vi "score sorter.vi"(11 "array of cluster":cluster{"Score":dbl, "Student ID":dbl}[](array[cluster])=[{"Score"=0.0, "Student ID"=1.0}, {"Score"=0.0, "Student ID"=2.0}, {"Score"=0.0, "Student ID"=3.0}, {"Score"=0.0, "Student ID"=4.0}, {"Score"=0.0, "Student ID"=5.0}, {"Score"=0.0, "Student ID"=6.0}, {"Score"=0.0, "Student ID"=7.0}, {"Score"=0.0, "Student ID"=8.0}, {"Score"=0.0, "Student ID"=9.0}, {"Score"=0.0, "Student ID"=10.0}, {"Score"=0.0, "Student ID"=11.0}, {"Score"=0.0, "Student ID"=12.0}, {"Score"=0.0, "Student ID"=13.0}, {"Score"=0.0, "Student ID"=14.0}, {"Score"=0.0, "Student ID"=15.0}, {"Score"=0.0, "Student ID"=16.0}, {"Score"=0.0, "Student ID"=17.0}, {"Score"=0.0, "Student ID"=18.0}, {"Score"=0.0, "Student ID"=19.0}, {"Score"=0.0, "Student ID"=20.0}, {"Score"=0.0, "Student ID"=21.0}, {"Score"=0.0, "Student ID"=22.0}, {"Score"=0.0, "Student ID"=23.0}, {"Score"=0.0, "Student ID"=24.0}, {"Score"=0.0, "Student ID"=25.0}, {"Score"=0.0, "Student ID"=26.0}, {"Score"=0.0, "Student ID"=27.0}, {"Score"=0.0, "Student ID"=28.0}, {"Score"=0.0, "Student ID"=29.0}, {"Score"=0.0, "Student ID"=30.0}, {"Score"=0.0, "Student ID"=31.0}, {"Score"=0.0, "Student ID"=32.0}, {"Score"=0.0, "Student ID"=33.0}, {"Score"=0.0, "Student ID"=34.0}, {"Score"=0.0, "Student ID"=35.0}, {"Score"=0.0, "Student ID"=36.0}, {"Score"=0.0, "Student ID"=37.0}, {"Score"=0.0, "Student ID"=38.0}, {"Score"=0.0, "Student ID"=39.0}, {"Score"=0.0, "Student ID"=40.0}, {"Score"=0.0, "Student ID"=41.0}, {"Score"=0.0, "Student ID"=42.0}, {"Score"=0.0, "Student ID"=43.0}, {"Score"=0.0, "Student ID"=44.0}, {"Score"=0.0, "Student ID"=45.0}, {"Score"=0.0, "Student ID"=46.0}, {"Score"=0.0, "Student ID"=47.0}, {"Score"=0.0, "Student ID"=48.0}, {"Score"=0.0, "Student ID"=49.0}, {"Score"=0.0, "Student ID"=50.0}]) -> (3 "sorted by score":cluster{"Score":dbl, "Student ID":dbl}[](array[cluster])=[{"Score"=0.0, "Student ID"=1.0}, {"Score"=0.0, "Student ID"=2.0}, {"Score"=0.0, "Student ID"=3.0}, {"Score"=0.0, "Student ID"=4.0}, {"Score"=0.0, "Student ID"=5.0}, {"Score"=0.0, "Student ID"=6.0}, {"Score"=0.0, "Student ID"=7.0}, {"Score"=0.0, "Student ID"=8.0}, {"Score"=0.0, "Student ID"=9.0}, {"Score"=0.0, "Student ID"=10.0}, {"Score"=0.0, "Student ID"=11.0}, {"Score"=0.0, "Student ID"=12.0}, {"Score"=0.0, "Student ID"=13.0}, {"Score"=0.0, "Student ID"=14.0}, {"Score"=0.0, "Student ID"=15.0}, {"Score"=0.0, "Student ID"=16.0}, {"Score"=0.0, "Student ID"=17.0}, {"Score"=0.0, "Student ID"=18.0}, {"Score"=0.0, "Student ID"=19.0}, {"Score"=0.0, "Student ID"=20.0}, {"Score"=0.0, "Student ID"=21.0}, {"Score"=0.0, "Student ID"=22.0}, {"Score"=0.0, "Student ID"=23.0}, {"Score"=0.0, "Student ID"=24.0}, {"Score"=0.0, "Student ID"=25.0}, {"Score"=0.0, "Student ID"=26.0}, {"Score"=0.0, "Student ID"=27.0}, {"Score"=0.0, "Student ID"=28.0}, {"Score"=0.0, "Student ID"=29.0}, {"Score"=0.0, "Student ID"=30.0}, {"Score"=0.0, "Student ID"=31.0}, {"Score"=0.0, "Student ID"=32.0}, {"Score"=0.0, "Student ID"=33.0}, {"Score"=0.0, "Student ID"=34.0}, {"Score"=0.0, "Student ID"=35.0}, {"Score"=0.0, "Student ID"=36.0}, {"Score"=0.0, "Student ID"=37.0}, {"Score"=0.0, "Student ID"=38.0}, {"Score"=0.0, "Student ID"=39.0}, {"Score"=0.0, "Student ID"=40.0}, {"Score"=0.0, "Student ID"=41.0}, {"Score"=0.0, "Student ID"=42.0}, {"Score"=0.0, "Student ID"=43.0}, {"Score"=0.0, "Student ID"=44.0}, {"Score"=0.0, "Student ID"=45.0}, {"Score"=0.0, "Student ID"=46.0}, {"Score"=0.0, "Student ID"=47.0}, {"Score"=0.0, "Student ID"=48.0}, {"Score"=0.0, "Student ID"=49.0}, {"Score"=0.0, "Student ID"=50.0}])   [LabVIEW 2014]
panel:
  out "index":i32[](array[numeric])
  out "Sorted Array":dbl[](array[numeric])
  out "swap":bool
  out "Index Sorted Array":dbl[](array[numeric])
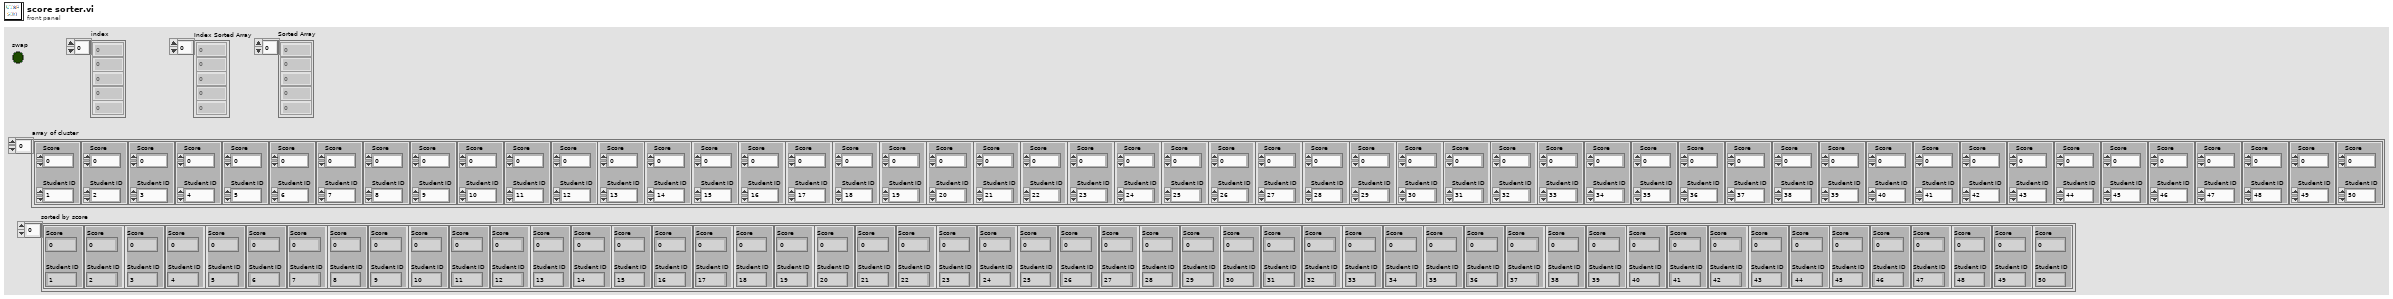
[diagram p1: front panel]
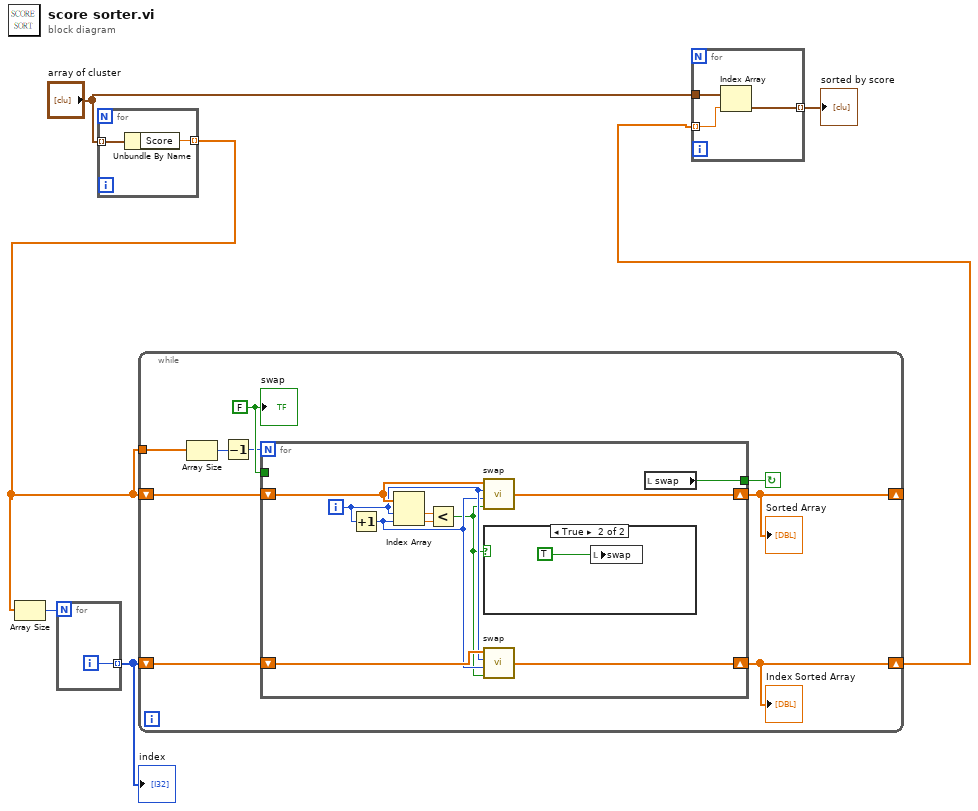
[diagram p0: block diagram]
diagram:
  n1 = for {
    tunnel: "array of cluster" -> [w8] mode=indexing
    tunnel: [w7] -> w2 mode=indexing
    n2 = Unbundle By Name(w8) -> ("Score"=w7:dbl)
  }
  n3 = Array Size(array=w2) -> (size(s)=w4:i32)
  n4 = for {
    N: w4 -> [_]
    tunnel: [w9] -> w3 mode=indexing
    i -> [w9]
  }
  "index" <- w3
  n5 = while {
    tunnel: w2 -> [w16]
    shift-right: [w15] -> _
    shift-left: w2 -> [w14]
    shift-right: [w10] -> w1
    shift-left: w3 -> [w11]
    stop <- w13 continue-if-true
    w17 = FALSE
    n6 = Array Size(array=w16) -> (size(s)=w18:i32)
    n7 = Decrement(x=w18) -> (x-1=w12:i32)
    n8 = for {
      N: w12 -> [_]
      shift-right: [w27] -> w15
      shift-left: w14 -> [w28]
      tunnel: w17 -> [_]
      tunnel: [w26] -> w13
      shift-right: [w22] -> w10
      shift-left: w11 -> [w25]
      i -> [w24]
      n9 = Increment(x=w24) -> (x+1=w23:i32)
      n10 = Index Array(array=w28, index #1=w24, index #2=w23) -> (element #1=w21:dbl, element #2=w20:dbl)
      n11 = Less?(x=w21, y=w20) -> (x < y?=w19:bool)
      n12 = call "swap.vi"("swap"=w19, "Index 2"=w23, "Index 1"=w24, "Array"=w28) -> ("Swapped Array"=w27:dbl[])
      n13 = case shown="True" w19 {
        frame False {
        }
        frame True {
          n14 = local write "swap"(TRUE) -> ()
        }
      }
      n15 = call "swap.vi"("swap"=w19, "Index 2"=w23, "Index 1"=w24, "Array"=w25) -> ("Swapped Array"=w22:dbl[])
      n16 = local read "swap"() -> (w26:bool)
    }
    "Sorted Array" <- w15
    "Index Sorted Array" <- w10
    "swap" <- w17
  }
  n17 = for {
    tunnel: w1 -> [w31] mode=indexing
    tunnel: "array of cluster" -> [w32]
    tunnel: [w30] -> w5 mode=indexing
    n18 = Index Array "Index Array"(array=w32, index=w31) -> (element=w30:cluster{"Score":dbl, "Student ID":dbl})
  }
  "sorted by score" <- w5
